vi "PH_PP_CurrentMeas.evt call Read DAQs.vi"(0 "i ref in":refnum<vi>, 2 "Instance name":string="N/A", 5 "error in (no error)":errorcluster) -> (14 "i ref out":refnum<vi>, 19 "error out":errorcluster)   [LabVIEW 2014, in "PH_PP_CurrentMeas.lvlib"]
doc: "This VI calls an event by a simple call."
uses:
  PH_PP_CurrentMeas.lvlib
  CS_Core/BaseProcess/BaseProcess.lvlib
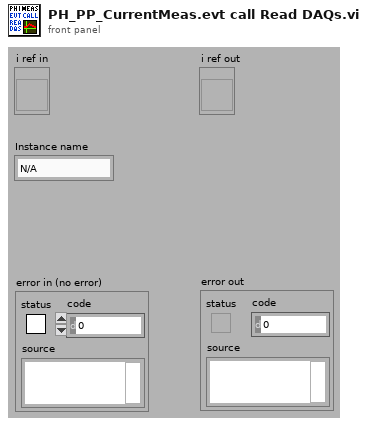
[diagram p1: front panel]
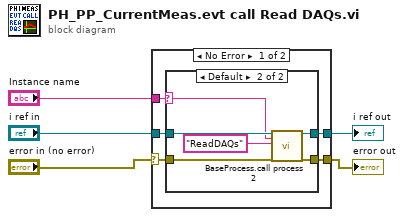
[diagram p0: block diagram]
diagram:
  n1 = case shown="No Error" "error in (no error)" {
    selector: "error in (no error)" -> [w6 w19]
    tunnel: "i ref in" -> [w10 w20]
    tunnel: [w9 w20] -> w4
    tunnel: [w8 w19] -> w3
    tunnel: "Instance name" -> [w7 _]
    frame No Error {
      n2 = case shown="Default" w7 {
        selector: w7 -> [_ w13]
        tunnel: w6 -> [w11 w17]
        tunnel: w10 -> [w12 w16]
        tunnel: [w12 w15] -> w9
        tunnel: [w11 w14] -> w8
        frame "N/A" {
        }
        frame Default {
          n3 = call "BaseProcess.call process 2.vi"("i ref in"=w16, "Object"=w13, "Selector"="ReadDAQs", "error in (no error)"=w17) -> ("i ref out"=w15:refnum<vi>, "error out"=w14:errorcluster)  [unwired: 14 in]
        }
      }
    }
    frame Error {
    }
  }
  "error out" <- w3
  "i ref out" <- w4
